vi "Calibrate Needle Tip.vi"(8 "error in":errorcluster, 11 "SyringeTool in":refnum<class "SyringeTool Class.lvclass">) -> (0 "error out":errorcluster, 3 "SyringeTool out":refnum<class "SyringeTool Class.lvclass">)   [LabVIEW 2011, in "SyringeTool Class.lvclass"]
uses:
  SyringeTool Class.lvclass
  Vec3d Class/Vec3d Class.lvclass
  WorkTable Class/WorkTable Class.lvclass
panel:
  out "Offset(mm)":cluster{"X":dbl, "Y":dbl, "Z":dbl}
  in  "Finished":bool
  in  "Camera Selection":enum32{"Radio Selection 1", "Radio Selection 2"}(radio)
  out "preview":T1(plugin-control)
  # "Use the MPG  hand control to\nmove the needle tip to the center\nof the image in both X and Y"
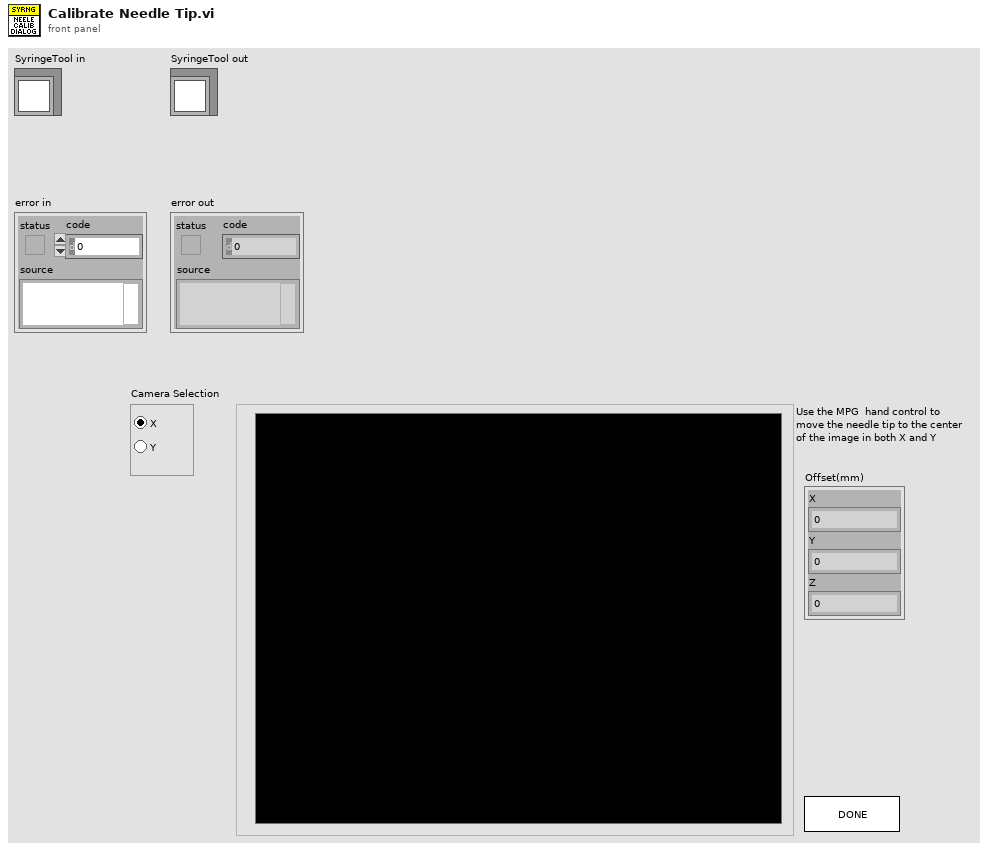
[diagram p1: front panel]
types:
  T1 = typedef "IMAQ Image.ctl" = refnum<image>
  T2 = typedef "Physical Image.ctl" = cluster{"Image Position":refnum<class "Vec3d Class.lvclass">, "Image Reference":T1, "Field of View":cluster{"x(mm)":dbl, "y(mm)":dbl}}
  T3 = typedef "Worktable_Syringe.ctl" = cluster{"Syringe Holder":enum16{"Empty", "Populated", "Calibrated"}, "Mixing Time":timestamp, "Tip Offset":refnum<class "Vec3d Class.lvclass">}
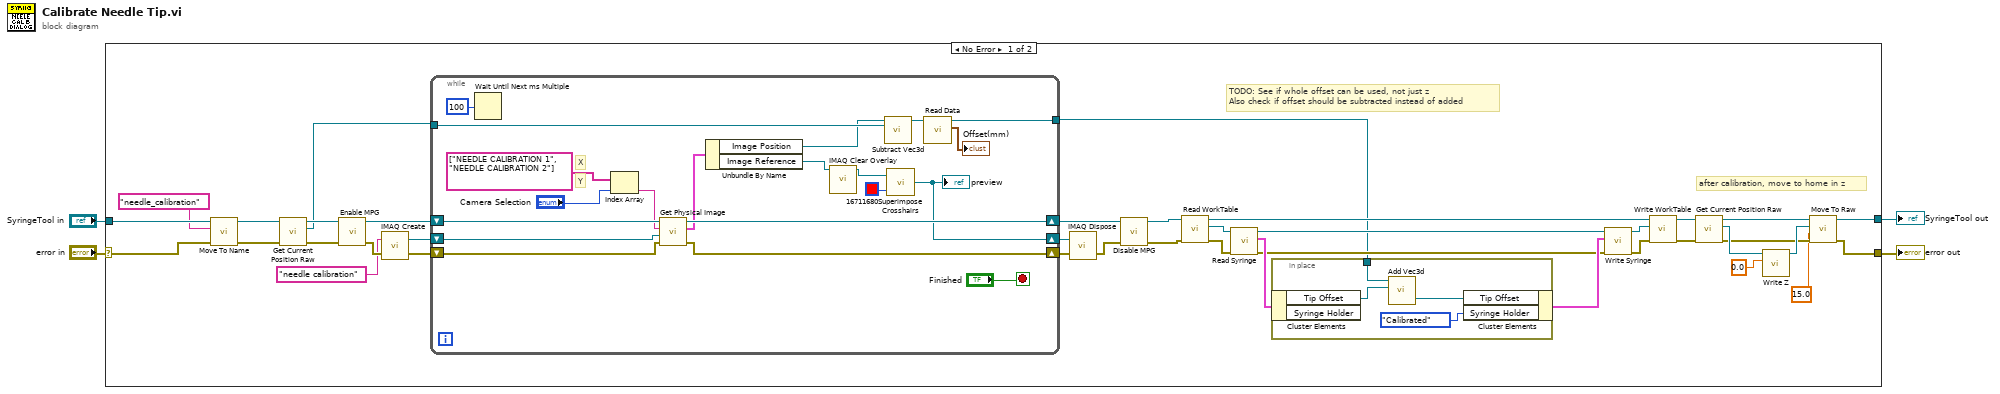
[diagram p0: block diagram]
diagram:
  n1 = case shown="No Error" "error in" {
    selector: "error in" -> [w24 w69]
    tunnel: [w11 w69] -> w3
    tunnel: [w12 w68] -> w1
    tunnel: "SyringeTool in" -> [w22 w68]
    frame No Error {
      # "after calibration, move to home in z"
      # "TODO: See if whole offset can be used, not just z\nAlso check if offset should be subtracted instead of added"
      n2 = call-dynamic "Move To Name.vi"("error in"=w24, "Destination Name"="needle_calibration", "Gantry in"=w22) -> ("error out"=w23:errorcluster, "Gantry out"=w21:refnum<class "SyringeTool Class.lvclass">)  [unwired: 7 in]
      n3 = call-dynamic "Get Current Position Raw.vi"("error in (no error)"=w23, "Gantry Class in"=w21) -> ("error out"=w37:errorcluster, "Vec3d Class out"=w35:refnum<class "Vec3d Class.lvclass">, "Gantry Class out"=w36:refnum<class "SyringeTool Class.lvclass">)  [unwired: 7 in]
      n4 = call-dynamic "Enable MPG.vi"("error in (no error)"=w37, "Gantry Class in"=w36) -> ("error out"=w42:errorcluster, "Gantry Class out"=w43:refnum<class "SyringeTool Class.lvclass">)  [unwired: 8 in]
      n5 = call "IMAQ Create"("Image Name"="needle calibration", "error in (no error)"=w42) -> ("New Image"=w40:T1, "error out"=w41:errorcluster)  [unwired: 3 in]
      n6 = while {
        shift-right: [w66] -> w8
        shift-left: w43 -> [w67]
        shift-right: [w51] -> w39
        shift-left: w40 -> [w65]
        shift-right: [w52] -> w38
        shift-left: w41 -> [w64]
        tunnel: w35 -> [w57]
        tunnel: [w54] -> w9
        stop <- "Finished" stop-if-true
        # "Y"
        # "X"
        n7 = Wait Until Next ms Multiple(millisecond multiple=100) -> ()  [unwired: 1 out]
        n8 = Index Array(array=string[] ["NEEDLE CALIBRATION 1", "NEEDLE CALIBRATION 2"], index="Camera Selection") -> (element=w61:string)
        n9 = call-dynamic "Get Physical Image.vi"("error in"=w64, "Image In"=w65, "Camera Name"=w61, "Gantry in"=w67) -> ("error out"=w52:errorcluster, "Physical Image"=w60:T2, "Gantry out"=w66:refnum<class "SyringeTool Class.lvclass">)  [unwired: 5 in]
        n10 = Unbundle By Name(w60) -> ("Image Position"=w56:refnum<class "Vec3d Class.lvclass">, "Image Reference"=w49:T1)
        n11 = call "IMAQ Clear Overlay"("Image"=w49) -> ("Image Out"=w48:T1)  [unwired: 9 in, 1 out]
        n12 = call "Subtract Vec3d.vi"("Vec3d in 2"=w57, "Vec3d in 1"=w56) -> ("Vec3d Class out"=w55:refnum<class "Vec3d Class.lvclass">)  [unwired: 8 in, 1 out]
        n13 = call "Superimpose Crosshairs.vi"("Grid Line Color"=u32 16711680, "Refnum in"=w48) -> ("Refnum out"=w51:T1)
        "preview" <- w51
        n14 = call-dynamic "Read Data.vi"("Vec3d Class in"=w55) -> ("Data"=→"Offset(mm)":cluster{"X":dbl, "Y":dbl, "Z":dbl}, "Vec3d Class out"=w54:refnum<class "Vec3d Class.lvclass">)  [unwired: 8 in, 1 out]
      }
      n15 = call "IMAQ Dispose"("Image"=w39, "error in (no error)"=w38) -> ("error out"=w6:errorcluster)  [unwired: 4 in]
      n16 = call-dynamic "Disable MPG.vi"("error in"=w6, "Gantry in"=w8) -> ("error out"=w5:errorcluster, "Gantry out"=w7:refnum<class "SyringeTool Class.lvclass">)  [unwired: 8 in]
      n17 = call-dynamic "Read WorkTable.vi"("error in"=w5, "Gantry Class in"=w7) -> ("error out"=w33:errorcluster, "WorkTable Class.lvclass"=w32:refnum<class "WorkTable Class.lvclass">, "Gantry Class out"=w28:refnum<class "SyringeTool Class.lvclass">)  [unwired: 7 in]
      n18 = call "Read Syringe.vi"("error in"=w33, "WorkTable in"=w32) -> ("error out"=w26:errorcluster, "Syringe"=w31:T3, "WorkTable out"=w29:refnum<class "WorkTable Class.lvclass">)  [unwired: 7 in]
      n19 = in-place {
        in-place-border: w9 -> [w44]
        n20 = in-place-cluster #1(w31) -> ("Tip Offset"=w45:refnum<class "Vec3d Class.lvclass">)  [unwired: 1 out]
        n21 = call-dynamic "Add Vec3d.vi"(10:"Vec3d Class in"=w45, 11:"Vec3d Class in"=w44) -> ("Vec3d Class out"=w46:refnum<class "Vec3d Class.lvclass">)  [unwired: 8 in, 1 out]
        n22 = in-place-cluster #1("Tip Offset"=w46, "Syringe Holder"=enum16{"Empty", "Populated", "Calibrated"}."Calibrated") -> (w30:T3)
      }
      n23 = call-dynamic "Write Syringe.vi"("error in (no error)"=w26, "Syringe"=w30, "WorkTable Class in"=w29) -> ("error out"=w25:errorcluster, "WorkTable Class out"=w27:refnum<class "WorkTable Class.lvclass">)  [unwired: 7 in]
      n24 = call-dynamic "Write WorkTable.vi"("error in (no error)"=w25, "WorkTable Class.lvclass"=w27, "Gantry Class in"=w28) -> ("error out"=w18:errorcluster, "Gantry Class out"=w19:refnum<class "SyringeTool Class.lvclass">)  [unwired: 7 in]
      n25 = call-dynamic "Get Current Position Raw.vi"("error in (no error)"=w18, "Gantry Class in"=w19) -> ("error out"=w13:errorcluster, "Vec3d Class out"=w17:refnum<class "Vec3d Class.lvclass">, "Gantry Class out"=w15:refnum<class "SyringeTool Class.lvclass">)  [unwired: 7 in]
      n26 = call-dynamic "Write Z.vi"("Z"=0.0, "Vec3d Class in"=w17) -> ("Vec3d Class out"=w14:refnum<class "Vec3d Class.lvclass">)  [unwired: 8 in, 1 out]
      n27 = call-dynamic "Move To Raw.vi"("error in"=w13, "Speed"=15.0, "Destination"=w14, "Gantry in"=w15) -> ("error out"=w11:errorcluster, "Gantry out"=w12:refnum<class "SyringeTool Class.lvclass">)  [unwired: 6 in]
    }
    frame Error {
    }
  }
  "error out" <- w3
  "SyringeTool out" <- w1
